vi "Userlist Message Callback.vi"(7 "Owner":refnum<class>, 11 "Message":refnum<class "Message.lvclass">) -> (0 "error out":errorcluster)   [LabVIEW 2020, in "LV Chat Client.lvclass"]
uses:
  LV Chat Client.lvclass
  <vilib>/IlluminatedG/lv-msg-simple/Stream-Simple-Msg/Message/Message.lvclass
  LV Chat Client.lvclass/LV Chat Client.ctl
  9460544c-6bf9-4dc1-88bc-113ddb7eadc4.vi
  <vilib>/IlluminatedG/lv-msg-simple/Stream-Simple-Msg/Message/Data and Type.vi
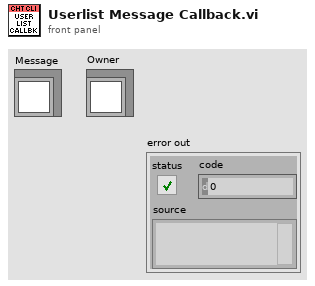
[diagram p1: front panel]
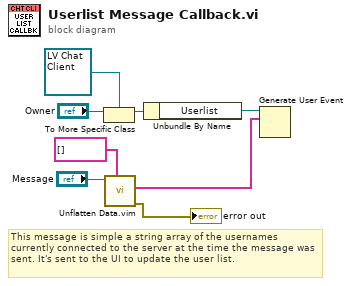
[diagram p0: block diagram]
diagram:
  # "This message is simple a string array of the usernames currently connected to the server at the time the message was sent. It's sent to the UI to update the user list."
  n1 = To More Specific Class(target class=refnum<class "LV Chat Client.lvclass"> refnum ("LV Chat Client.lvclass"), reference="Owner") -> (specific class reference=w5:refnum<class "LV Chat Client.lvclass">)  [unwired: 1 in, 1 out]
  n2 = call "Unflatten Data.vim"("Data Type (String)"=string[] [], "Message in"="Message") -> ("error out"=→"error out":errorcluster, "Unflattened Data"=w3:string[])  [unwired: 7 in, 1 out]
  n3 = Unbundle By Name(w5) -> ("Userlist"=w4:refnum<user-event>)
  n4 = Generate User Event(user event=w4, event data cluster=w3) -> ()  [unwired: 2 in, 2 out]
